vi "2 Runprotect.vi"(10 "Wind Records":dbl[][](array[numeric])) -> ()   [LabVIEW 2011]
doc: "This VI is launched, when the Runprotect Boolean in the Wind Records VI is activated.\nIt calculates a Wind Direction and a Windspeed out of the REcords that were taken before.\nIn this calculations, the newer values are counted higher than older values.\nThe calculated values are absolute values and we use the VI \"1 Wind Calculator\" from the Simulation Platform to calculate the Apparent Wind."
uses:
  2 Globals/2 Global.vi
  <vilib>/gmath/NI_Gmath.lvlib
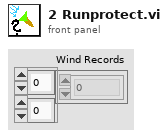
[diagram p1: front panel]
types:
  T1 = typedef "heading.ctl" = dbl
  T2 = typedef "robot velocity.ctl" = cluster{"East":dbl, "North":dbl}
  T3 = typedef "apparent wind speed.ctl" = dbl
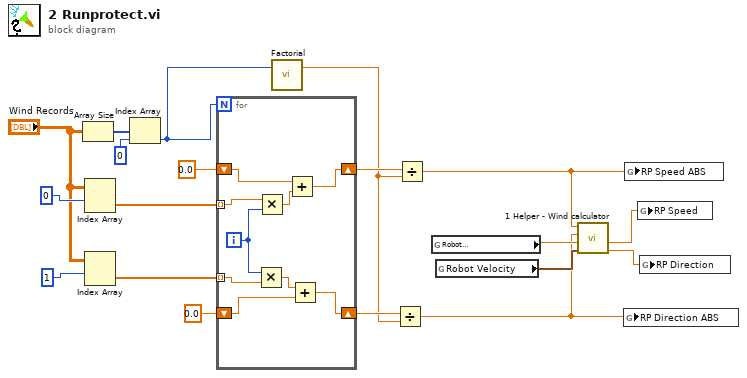
[diagram p0: block diagram]
diagram:
  n1 = Array Size(array="Wind Records") -> (size(s)=w18:i32[])
  n2 = Index Array(array="Wind Records", index (row)=0) -> (element=w14:dbl[])  [unwired: 1 in]
  n3 = Index Array(array="Wind Records", index (row)=1) -> (element=w13:dbl[])  [unwired: 1 in]
  n4 = Index Array(array=w18, index=0) -> (element=w17:i32)
  n5 = for {
    N: w17 -> [_]
    tunnel: w14 -> [w27] mode=indexing
    tunnel: w13 -> [w26] mode=indexing
    shift-right: [w21] -> w10
    shift-left: 0.0 -> [w25]
    shift-right: [w20] -> w9
    shift-left: 0.0 -> [w22]
    i -> [w28]
    n6 = Multiply(x=w28, y=w26) -> (x*y=w23:dbl)
    n7 = Multiply(x=w27, y=w28) -> (x*y=w24:dbl)
    n8 = Add(x=w25, y=w24) -> (x+y=w21:dbl)
    n9 = Add(x=w23, y=w22) -> (x+y=w20:dbl)
  }
  n10 = call <vilib>:"Factorial.vi"("n"=w17) -> ("n!"=w8:dbl)  [unwired: 2 in]
  n11 = Divide(x=w9, y=w8) -> (x/y=w1:dbl)
  n12 = Divide(x=w10, y=w8) -> (x/y=w2:dbl)
  n13 = global read "2 Global.vi" "Robot\nHeading"() -> (w6:T1)
  n14 = global read "2 Global.vi" "Robot Velocity"() -> (w5:T2)
  n15 = call "1 Helper - Wind calculator.vi"("Robot Velocity"=w5, "Heading"=w6, "Absolute Wind Direction"=w1, "Absolute Wind Speed"=w2) -> ("Apparent Wind Direction"=w3:T1, "Apparent Wind Speed"=w4:T3)  [unwired: 4 in, 2 out]
  n16 = global write "2 Global.vi" "RP Direction ABS"(w1) -> ()
  n17 = global write "2 Global.vi" "RP Speed ABS"(w2) -> ()
  n18 = global write "2 Global.vi" "RP Speed"(w4) -> ()
  n19 = global write "2 Global.vi" "RP Direction"(w3) -> ()
